vi "Read connect timeout.vi"(8 "error in (no error)":errorcluster, 11 "TCP in":refnum<class "TCP.lvclass">) -> (0 "error out":errorcluster, 2 "connect timeout":i32=502, 3 "TCP out":refnum<class "TCP.lvclass">)   [LabVIEW 2019, in "TCP.lvclass"]
uses:
  TCP.lvclass
  TCP.lvclass/TCP.ctl
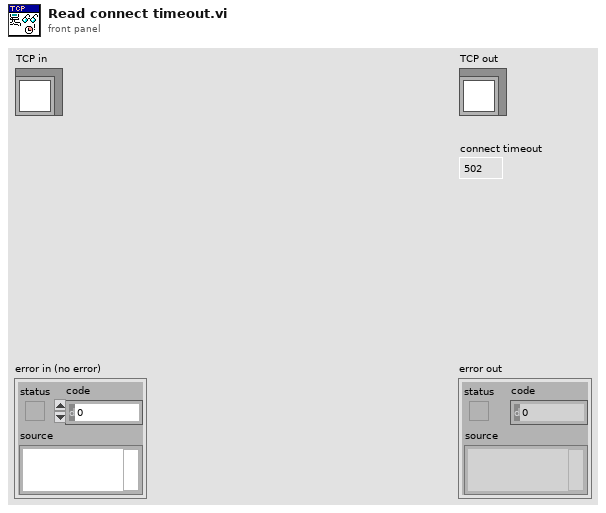
[diagram p1: front panel]
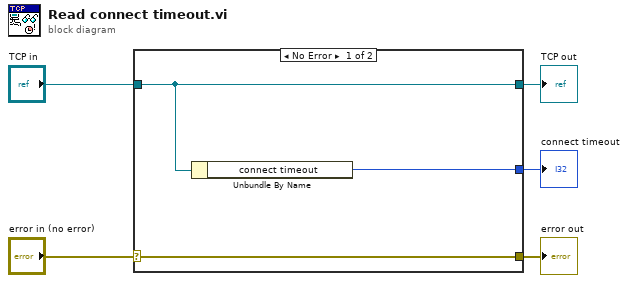
[diagram p0: block diagram]
diagram:
  n1 = case shown="No Error" "error in (no error)" {
    selector: "error in (no error)" -> [w8 w9]
    tunnel: [w8 w9] -> w4
    tunnel: [w7 w10] -> w2
    tunnel: "TCP in" -> [w7 w10]
    tunnel: [w6 _] -> w1
    frame No Error {
      n2 = Unbundle By Name(w7) -> ("connect timeout"=w6:i32)
    }
    frame Error {
    }
  }
  "error out" <- w4
  "TCP out" <- w2
  "connect timeout" <- w1
